vi "NewtonsPSM_Trim.vi"(7 "AC Level (1)":dbl=1.0 min=0.0 max=10.0 step=0.0001, 8 "error in":errorcluster, 9 "Tolerance (10)":dbl=10.0 min=0.0 max=100.0 step=0.01, 10 "AC Trim Data (Disabled)":enum16{"DISABLED", "CH1", "CH2"}(ring), 11 "VISA.name":refnum<visa-resource-name>) -> (0 "error out":errorcluster, 3 "VISA.name out":refnum<visa-resource-name>)   [LabVIEW 2025, in "NewtonsPSM1735.lvlib"]
doc: "This VI set the settings for wiring the PPA2530"
uses:
  NewtonsPSM1735.lvlib
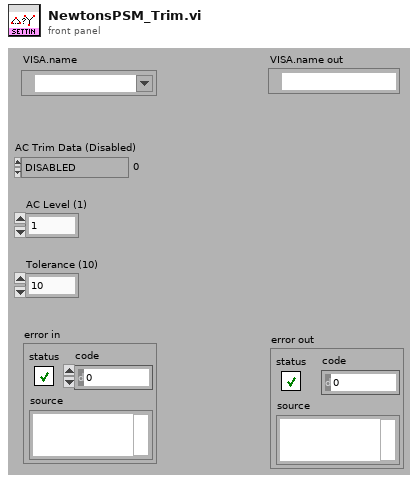
[diagram p1: front panel]
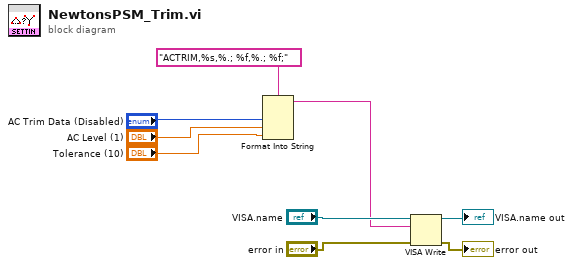
[diagram p0: block diagram]
diagram:
  n1 = Format Into String(format string="ACTRIM,%s,%.; %f,%.; %f;" ("chaîne de format"), "AC Trim Data (Disabled)", "AC Level (1)", "Tolerance (10)") -> (resulting string=w1:string)  [unwired: 2 in, 1 out]
  n2 = VISA Write(VISA resource name="VISA.name", write buffer=w1, error in (no error)="error in") -> (VISA resource name out=→"VISA.name out":refnum<visa-resource-name>, error out=→"error out":errorcluster)  [unwired: 1 out]
